vi "Left Heel Strike Detector.vi"(8 "Force Rate Threshold":dbl, 9 "Force Threshold":dbl, 11 "Sensors":T1) -> (0 "Heel State":i32, 1 "d_F":dbl, 2 "F":dbl, 3 "Heel Strike?":bool, 4 "error out":errorcluster)   [LabVIEW 2018]
uses:
  Sensor Data.ctl
  <vilib>/Analysis/3filter.llb/Filter Passband Type.ctl
  <vilib>/ptbypt/NI_PtbyPt.lvlib
  <vilib>/Analysis/NI_AALBase.lvlib
panel:
  out "fc":dbl
  out "fs":dbl
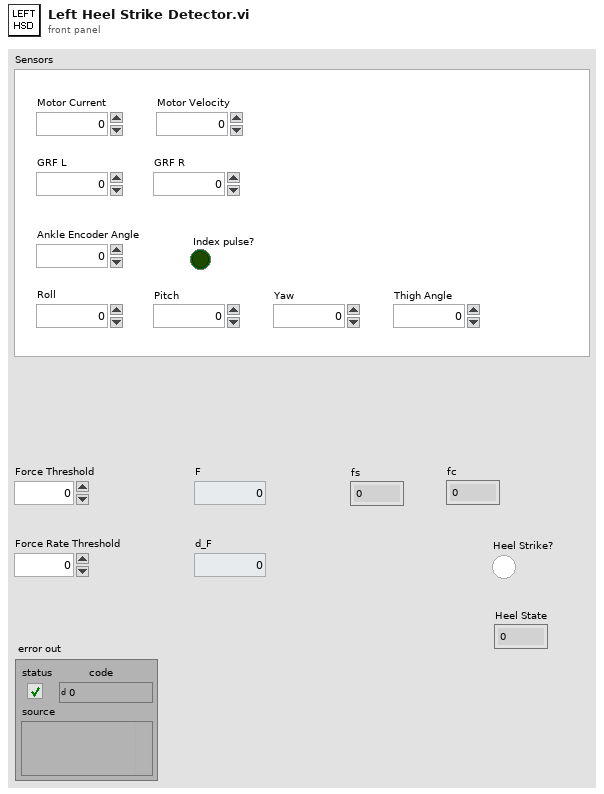
[diagram p1: front panel]
types:
  T1 = typedef "Sensor Data.ctl" = cluster{"Motor Current":dbl, "Motor Velocity":dbl, "Ankle Encoder Angle":dbl, "GRF L":dbl, "GRF R":dbl, "Index pulse?":bool, "Roll":dbl, "Pitch":dbl, "Yaw":dbl, "Thigh Angle":dbl}
  T2 = typedef "NI_AALBase.lvlib/Filter Passband Type.ctl" = enum32{"Lowpass", "Highpass", "Bandpass", "Bandstop"}
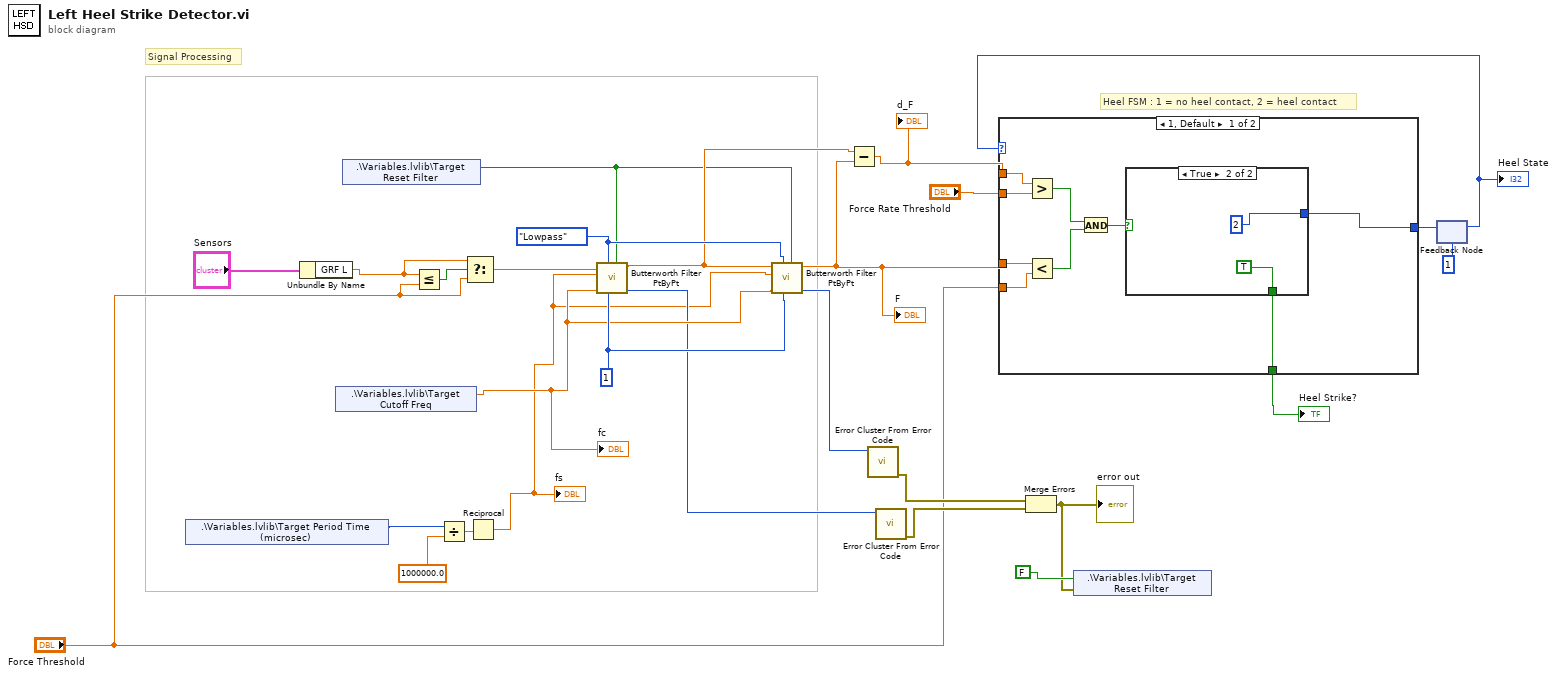
[diagram p0: block diagram]
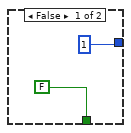
[diagram p2: hidden frame]
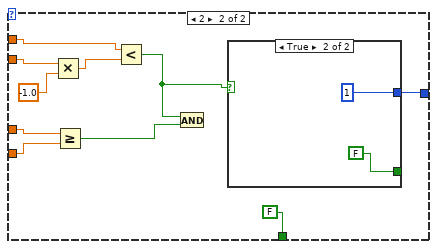
[diagram p3: hidden frame]
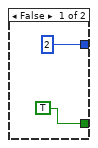
[diagram p4: hidden frame]
diagram:
  w25 = Filter_Passband_Type."Lowpass" ("filter type")
  w26 = 1 ("order")
  # "Signal Processing"
  # "Heel FSM : 1 = no heel contact, 2 = heel contact"
  n1 = shared-variable ".\\Variables.lvlib\\Target Period Time (microsec)"() -> (w16:u16)  [unwired: 1 in, 1 out]
  n2 = Unbundle By Name("Sensors") -> ("GRF L"=w6:dbl)
  n3 = shared-variable ".\\Variables.lvlib\\Target Cutoff Freq"() -> (w15:dbl)  [unwired: 1 in, 1 out]
  "fc" <- w15
  n4 = shared-variable ".\\Variables.lvlib\\Target Reset Filter"() -> (w3:bool)  [unwired: 1 in, 1 out]
  n5 = Less Or Equal?(x=w6, y="Force Threshold") -> (x <= y?=w7:bool)
  n6 = Divide(x=w16, y=1000000.0) -> (x/y=w24:dbl)
  n7 = Select(t=w6, s=w7, f="Force Threshold") -> (s? t:f=w4:dbl)
  n8 = Reciprocal(x=w24) -> (1/x=w8:dbl)
  "fs" <- w8
  n9 = call <vilib>:"Butterworth Filter PtByPt.vi"("initialize"=w3, "order"=w26, "filter type"=w25, "low cutoff freq: fl"=w15, "sampling freq: fs"=w8, "x"=w4) -> ("error"=w13:i32, "Filtered x"=w10:dbl)  [unwired: 3 in]
  n10 = call <vilib>:"Butterworth Filter PtByPt.vi"("initialize"=w3, "order"=w26, "filter type"=w25, "low cutoff freq: fl"=w15, "sampling freq: fs"=w8, "x"=w10) -> ("error"=w14:i32, "Filtered x"=w9:dbl)  [unwired: 3 in]
  "F" <- w9
  n11 = Subtract(x=w10, y=w9) -> (x-y=w18:dbl)
  "d_F" <- w18
  n12 = call <vilib>:"Error Cluster From Error Code.vi"("error code (0)"=w14) -> ("error out"=w12:errorcluster)  [unwired: 8 in]
  n13 = call <vilib>:"Error Cluster From Error Code.vi"("error code (0)"=w13) -> ("error out"=w11:errorcluster)  [unwired: 8 in]
  n14 = Merge Errors(w12, w11) -> (w1:errorcluster)
  "error out" <- w1
  n15 = shared-variable ".\\Variables.lvlib\\Target Reset Filter"(FALSE, error in=w1) -> ()  [unwired: 1 out]
  n16 = feedback #1(1) -> (w21:i32)
  "Heel State" <- w21
  n17 = case shown="1, Default" w21 {
    tunnel: [w35 w43] -> w20
    tunnel: [w34 FALSE] -> w17
    tunnel: "Force Rate Threshold" -> [w33 w48]
    tunnel: w18 -> [w32 w46]
    tunnel: w9 -> [w30 w50]
    tunnel: "Force Threshold" -> [w28 w49]
    frame 1, Default {
      n18 = Greater?(x=w32, y=w33) -> (0:w31:bool)
      n19 = Less?(x=w30, y=w28) -> (x < y?=w29:bool)
      n20 = And(x=w31, y=w29) -> (x .and. y?=w36:bool)
      n21 = case shown="True" w36 {
        tunnel: [1 2] -> w35
        tunnel: [FALSE TRUE] -> w34
        frame False {
        }
        frame True {
        }
      }
    }
    frame 2 {
      n22 = Multiply(x=w48, y=-1.0) -> (x*y=w45:dbl)
      n23 = Greater Or Equal?(x=w50, y=w49) -> (x >= y?=w44:bool)
      n24 = Less?(x=w46, y=w45) -> (x < y?=w41:bool)
      n25 = And(x=w41, y=w44) -> ()  [unwired: 1 out]
      n26 = case shown="True" w41 {
        tunnel: [2 1] -> w43
        tunnel: [TRUE FALSE] -> _
        frame False {
        }
        frame True {
        }
      }
    }
  }
  "Heel Strike?" <- w17
  n27 = feedback-in #1(w20) -> ()
